vi "Apply New DataTable.vi"(6 "Images Path":path, 8 "error in (no error)":errorcluster, 9 "DataArray":string[][](array[string]), 10 "ColumnSetup":T1[](array[typedef]) {"MinWidth" min=2 step=1; "AutoSizeMode" items=["None"=1, "ColumnHeader"=2, "AllCellsExceptHeader"=4, "AllCells"=6, "DisplayedCellsExceptHeader"=8, "DisplayedCells"=10, "Fill"=16]; "FillWeight" min=1 max=100}, 11 "DataGridView in":refnum<class "DataGridView.lvclass">) -> (0 "error out":errorcluster, 3 "DataGridView out":refnum<class "DataGridView.lvclass">)   [LabVIEW 2016, in "DataGrid.lvlib" / "DataGridView.lvclass"]
uses:
  <userlib>/LabVIEWdotNetDataGrid/source/DataGridView/DataGridView.lvclass
  <userlib>/LabVIEWdotNetDataGrid/source/GridColumn/ColumnDefinition.ctl
  <userlib>/LabVIEWdotNetDataGrid/source/GridColumn/ColumnType.ctl
  <userlib>/LabVIEWdotNetDataGrid/source/DataGridView/DataGridView.lvclass/DataGridView.ctl
  System.Windows.Forms
  <userlib>/LabVIEWdotNetDataGrid/source/DataGridView/Properties/Read DataGridView.vi
  <userlib>/LabVIEWdotNetDataGrid/source/DataTable/Add Rows (String).vi
  <userlib>/LabVIEWdotNetDataGrid/source/DataTable/DataTable.lvclass
  <userlib>/LabVIEWdotNetDataGrid/source/GridColumn/GridColumn.lvclass
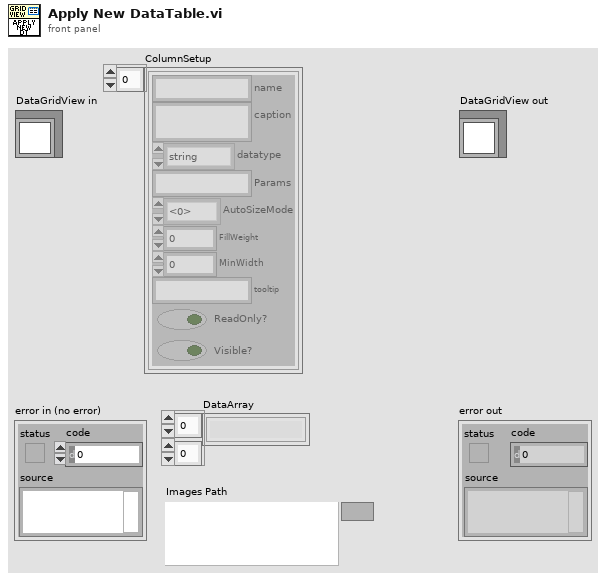
[diagram p1: front panel]
types:
  T1 = typedef "DataGrid.lvlib/GridColumn.lvclass/ColumnDefinition.ctl" = cluster{"name":string, "caption":string, "datatype":T2, "Params":string, "AutoSizeMode":i32, "FillWeight":sgl, "MinWidth":u32, "tooltip":string, "ReadOnly?":bool, "Visible?":bool}
  T2 = typedef "DataGrid.lvlib/GridColumn.lvclass/ColumnType.ctl" = enum16{"string", "image", "check", "numeric", "timestamp", "button", "combo", "link"}
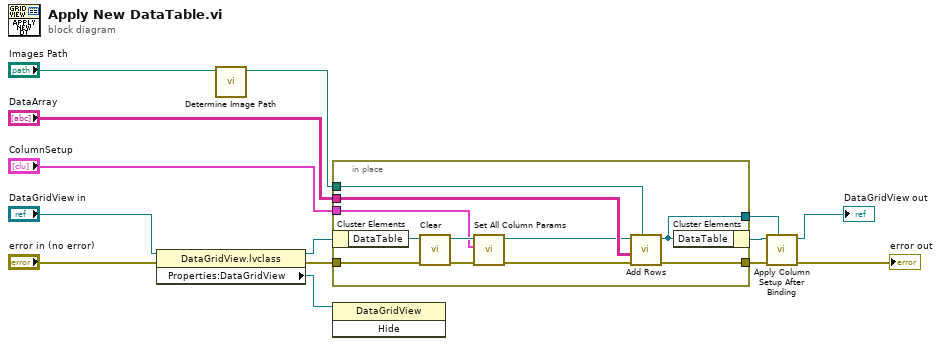
[diagram p0: block diagram]
diagram:
  n1 = property class="DataGridView.lvclass"(reference="DataGridView in", error in="error in (no error)") -> (reference out=w2:refnum<class "DataGridView.lvclass">, error out=w4:errorcluster, "Properties:DataGridView"=w1:refnum<k24>)
  n2 = call <userlib>:"Determine Image Path.vi"("image path"="Images Path") -> ("Path"=w8:path)  [unwired: 10 in]
  n3 = in-place {
    in-place-border: "ColumnSetup" -> [w15]
    in-place-border: "DataArray" -> [w24]
    in-place-border: w8 -> [w23]
    in-place-border: w4 -> [w22]
    in-place-border: [w20] -> w6
    in-place-border: [w19] -> w5
    n4 = in-place-cluster #1(w2) -> ("DataTable"=w25:refnum<class "DataTable.lvclass">)
    n5 = call <userlib>:"Clear.vi"("error in (no error)"=w22, "DataTable in"=w25) -> ("error out"=w21:errorcluster, "DataTable out"=w17:refnum<class "DataTable.lvclass">)  [unwired: 8 in]
    n6 = call <userlib>:"Set All Column Params.vi"("error in (no error)"=w21, "ColumnSetup"=w15, "DataTable in"=w17) -> ("error out"=w18:errorcluster, "DataTable out"=w16:refnum<class "DataTable.lvclass">)  [unwired: 7 in]
    n7 = call-poly <userlib>:"Add Rows.vi"("image path"=w23, "error in (no error)"=w18, "String Data"=w24, "DataTable in"=w16) -> ("error out"=w20:errorcluster, "DataTable out"=w19:refnum<class "DataTable.lvclass">)  [unwired: 6 in]
    n8 = in-place-cluster #1("DataTable"=w19) -> (w11:refnum<class "DataGridView.lvclass">)
  }
  n9 = invoke class="DataGridView" method="Hide"(reference=w1) -> ()  [unwired: 2 in, 3 out]
  n10 = call <userlib>:"Apply Column Setup After Binding.vi"("DataTable"=w5, "error in (no error)"=w6, "DataGridView in"=w11) -> ("error out"=→"error out":errorcluster, "DataGridView out"=→"DataGridView out":refnum<class "DataGridView.lvclass">)  [unwired: 7 in]
